vi "Get Terminals.vi"(8 "error in":errorcluster, 11 "id":string) -> (0 "error out":errorcluster, 3 "Terminals":refnum<vi>[](array[refnum]))   [LabVIEW 2026, in "G-AI Core.lvlib"]
uses:
  G-AI Core.lvlib
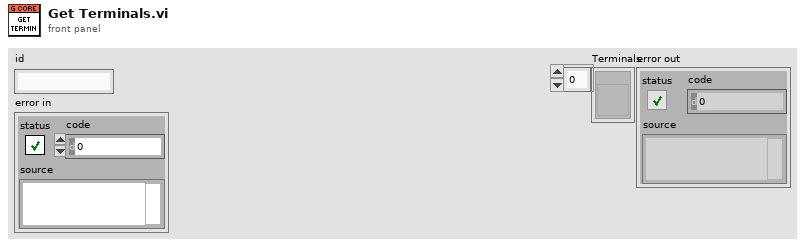
[diagram p1: front panel]
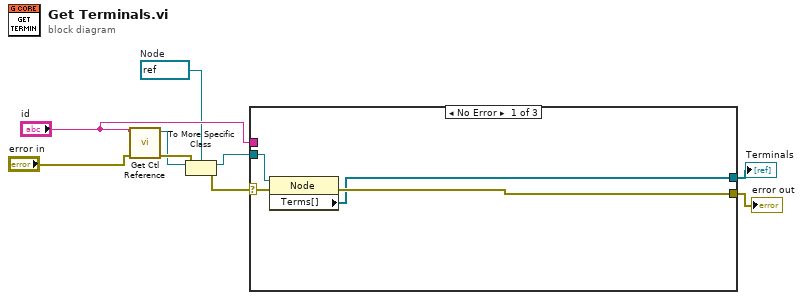
[diagram p0: block diagram]
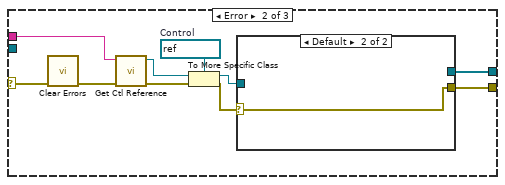
[diagram p2: hidden frame]
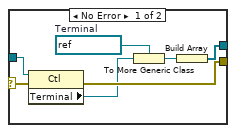
[diagram p3: hidden frame]
diagram:
  w3 = refnum<vi> refnum  # Node
  n1 = call "Get Ctl Reference.vi"("error in"="error in", "id"="id") -> ("error out"=w8:errorcluster, "ctl reference"=w5:refnum<vi>)  [unwired: 8 in]
  n2 = To More Specific Class(target class=w3, reference=w5, error in=w8) -> (specific class reference=w4:refnum<vi>, error out=w6:errorcluster)
  n3 = case shown="No Error" w6 {
    selector: w6 -> [w10 w23 w32]
    tunnel: [w13 w22 w32] -> w1
    tunnel: w4 -> [w12 _ _]
    tunnel: [w11 w21 _] -> w2
    tunnel: "id" -> [_ w18 _]
    frame No Error {
      n4 = property class="Node"(reference=w12, error in=w10) -> (error out=w13:errorcluster, "Terms[]"=w11:refnum<vi>[])  [unwired: 1 out]
    }
    frame Error {
      w14 = refnum<vi> refnum  # Control
      n5 = call <vilib>:"Clear Errors.vi"("error in (no error)"=w23) -> ("error out"=w20:errorcluster)  [unwired: 5 in, 1 out]
      n6 = call "Get Ctl Reference.vi"("error in"=w20, "id"=w18) -> ("error out"=w19:errorcluster, "ctl reference"=w16:refnum<vi>)  [unwired: 8 in]
      n7 = To More Specific Class(target class=w14, reference=w16, error in=w19) -> (specific class reference=w15:refnum<vi>, error out=w17:errorcluster)
      n8 = case shown="Default" w17 {
        selector: w17 -> [w26 w31]
        tunnel: [w30 w31] -> w22
        tunnel: w15 -> [w29 _]
        tunnel: [w27 _] -> w21
        frame No Error {
          w24 = refnum<vi> refnum  # Terminal
          n9 = property class="Ctl"(reference=w29, error in=w26) -> (error out=w30:errorcluster, "Terminal"=w28:refnum<vi>)  [unwired: 1 out]
          n10 = To More Generic Class(target class=w24, reference=w28) -> (generic class reference=w25:refnum<vi>)
          n11 = Build Array(w25) -> (w27:refnum<vi>[])
        }
        frame Default {
        }
      }
    }
    frame Default {
    }
  }
  "Terminals" <- w2
  "error out" <- w1
